vi "tree for Hardware Device Subpanel.vi"(1 "Data Types":T2(array[cluster]), 2 "Array":string[](array[string])=["Ring", "Elements", "to choose"], 3 "Data Names&Defaults":string[][](array[string])) -> (0 "Data Names&Data":string[][](array[string]))   [LabVIEW 2016, in "TSPopup.lvlib"]
doc: "Demo showing dynamically changing data types and working with a tree.\n\nType Sensitive Popup \nCopyright © 2007, J. David Saunders\nAll rights reserved."
uses:
  <userlib>/TSPopup/TSPopup.lvlib
  <userlib>/TSPopup/TSPopup.Popup Cluster.ctl
  <userlib>/TSPopup/TSPopup.lvclass
panel:
  in  "Array 2":string[](array[string])=["Ring", "Elements", "to choose"]
  in  "Remove Button":bool
  in  "Add Button":bool
  in  "Popups":T1 {"Boolean" items=["False", "True"]; "Ring" items=["Ring", "Elements", "to choose"]}
  in  "Cancel Button":bool
  in  "OK Button":bool
  in  "Data List":string(tree)
  # "Type Sensitive Popup \nCopyright © 2007, J. David Saunders\nAll rights reserved."
  # "Type Sensitive\nPopup"
  # "Boolean Colors"
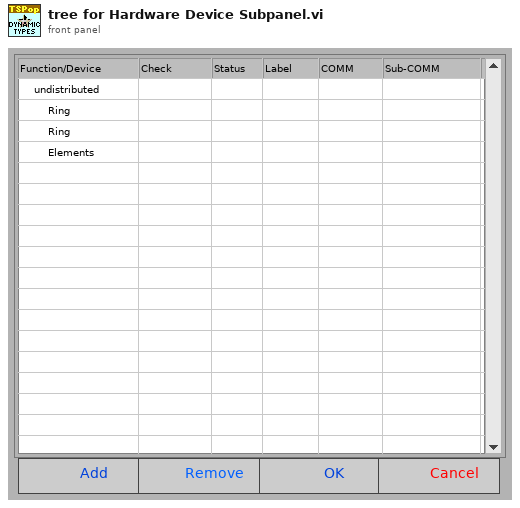
[diagram p1: front panel]
types:
  T1 = typedef "TSPopup.lvlib/TSPopup.lvclass/TSPopup.Popup Cluster.ctl" = cluster{"Unknown":bool, "Unknown 2":bool, "String":string, "Integer":i32, "Float":dbl, "Color":u32, "Boolean":u32, "Ring":u32, "Captioned String":cluster{"String":string, "OK":bool, "Cancel":bool}, "Captioned Integer":cluster{"First":i32, "OK":bool, "Cancel":bool}, "Boolean Colors":cluster{"False":cluster{"FG":u32, "BG":u32}, "True":cluster{"FG":u32, "BG":u32}, "T  to  F":cluster{"FG":u32, "BG":u32}, "F  to  T":cluster{"FG":u32, "BG":u32}, "OK":bool, "Cancel":bool}, "2-Int Cluster":cluster{"First":i32, "Second":i32, "OK":bool, "Cancel":bool}, "4-Int Cluster":cluster{"First":i32, "Second":i32, "Third":i32, "Fourth":i32, "OK":bool, "Cancel":bool}, "check":bool}
  T2 = cluster{"Data Type":string, "Caption/Ring Strings":string[]}[]
  T3 = typedef "LVPoint32TypeDef.ctl" = cluster{"Horizontal":i32, "Vertical":i32}
  T4 = typedef "TSPopup.lvlib/TSPopup.lvclass/TSPopup.Grid.Cell Info.ctl" = cluster{"Tag":string, "Row":i32, "Column":i32, "In Symbol?":bool, "In Data?":bool, "Cell String":string, "Ctl Refnum":refnum<vi>, "Prop Type":T5, "Ring Strings":string[]}
  T5 = typedef "TSPopup.lvlib/TSPopup.lvclass/TSPopup.Data Type.ctl" = enum16{"Unkown", "NO POPUP", "String", "Integer", "Float", "Color", "Boolean", "Ring", "Captioned String", "Captioned Integer", "Button Color", "2 Int Cluster", "4 Int Cluster", "check"}
  T6 = typedef "TSPopup.lvlib/TSPopup.lvclass/TSPopup.Popup Call Parameters.ctl" = cluster{"Prop Type":T5, "Initial Value":variant, "Caption Strings":string[], "Ring Strings":string[], "Cell Rect":cluster{"left":i16, "top":i16, "right":i16, "bottom":i16}, "Mouse Coords":cluster{"x":i16, "y":i16}, "Call Data":variant}
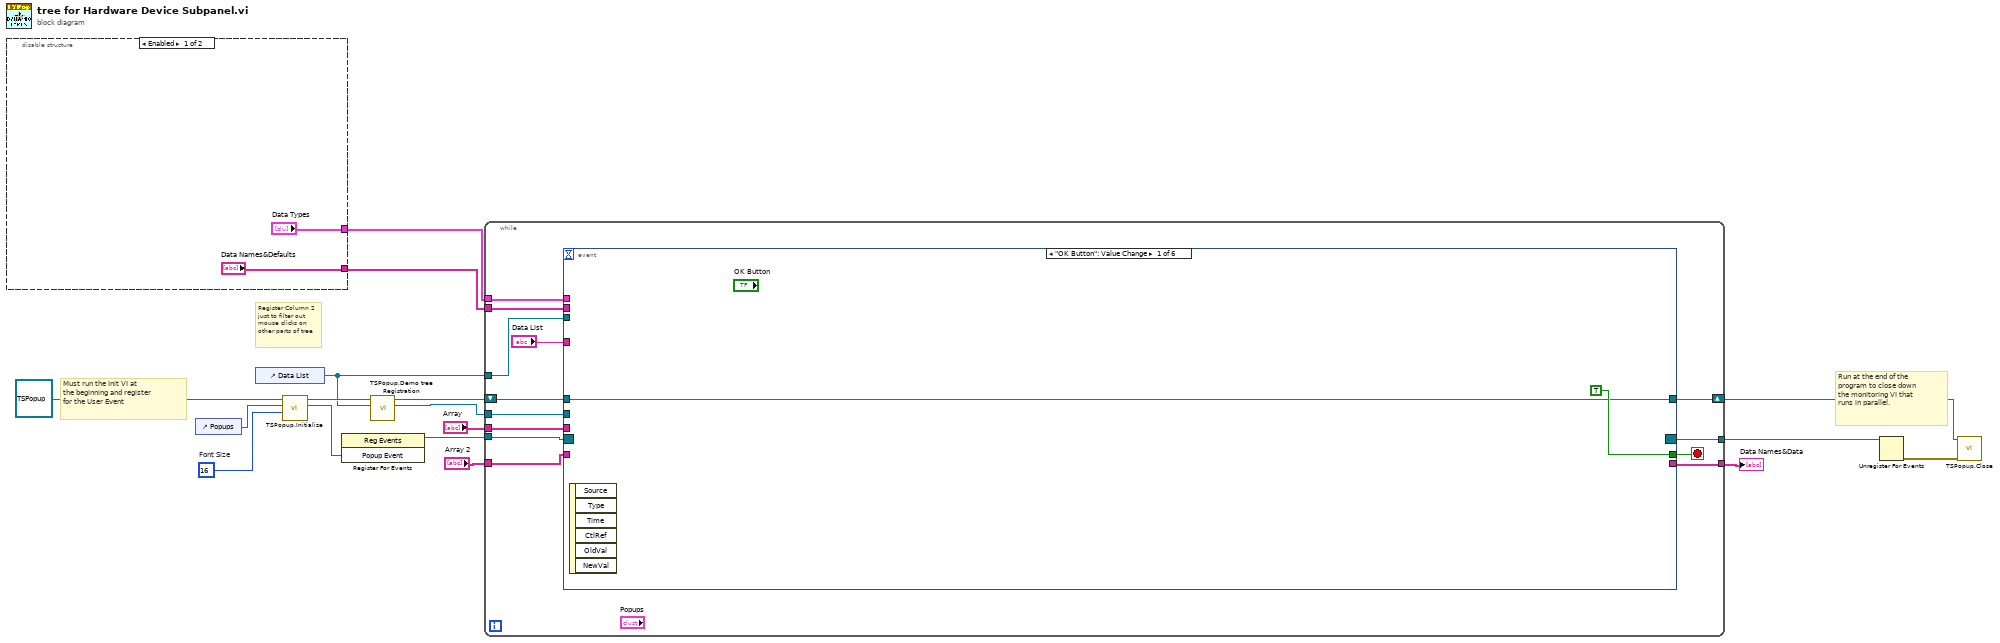
[diagram p0: block diagram]
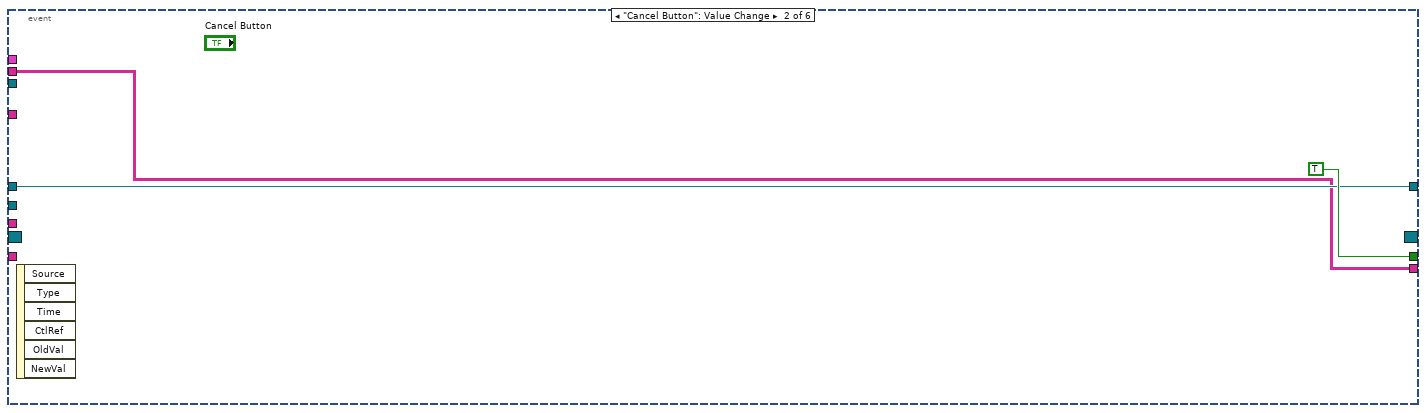
[diagram p2: hidden frame]
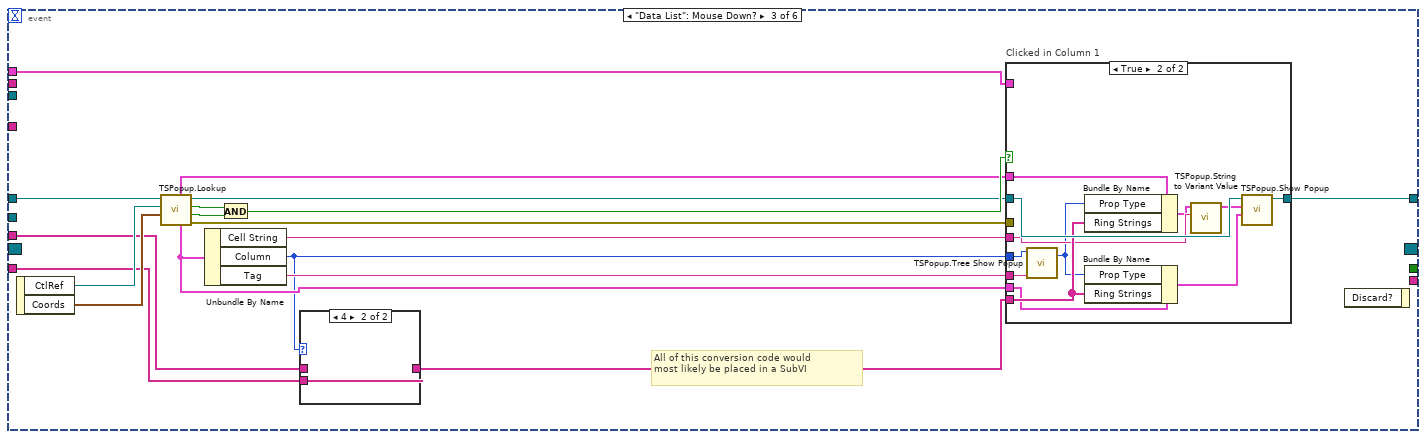
[diagram p3: hidden frame]
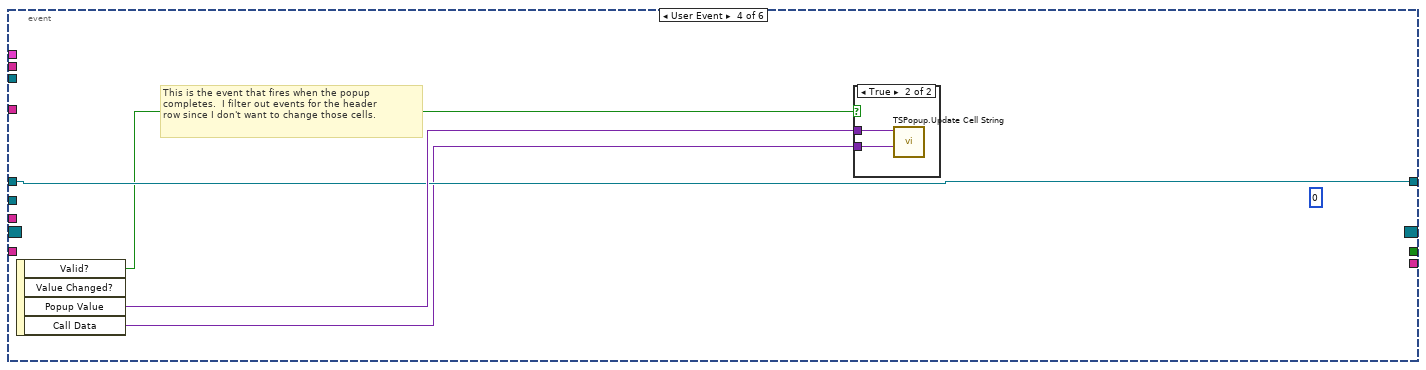
[diagram p6: hidden frame]
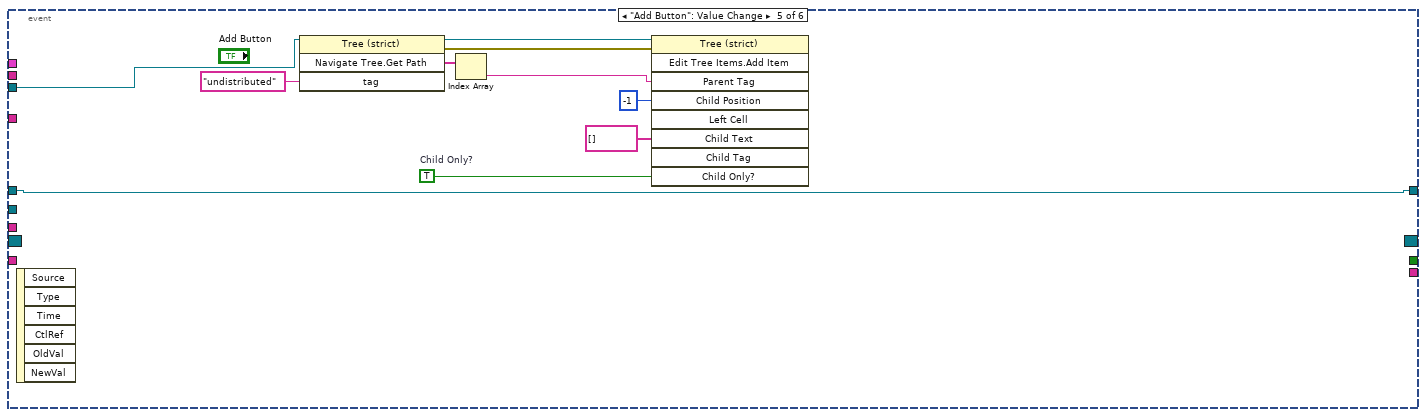
[diagram p8: hidden frame]
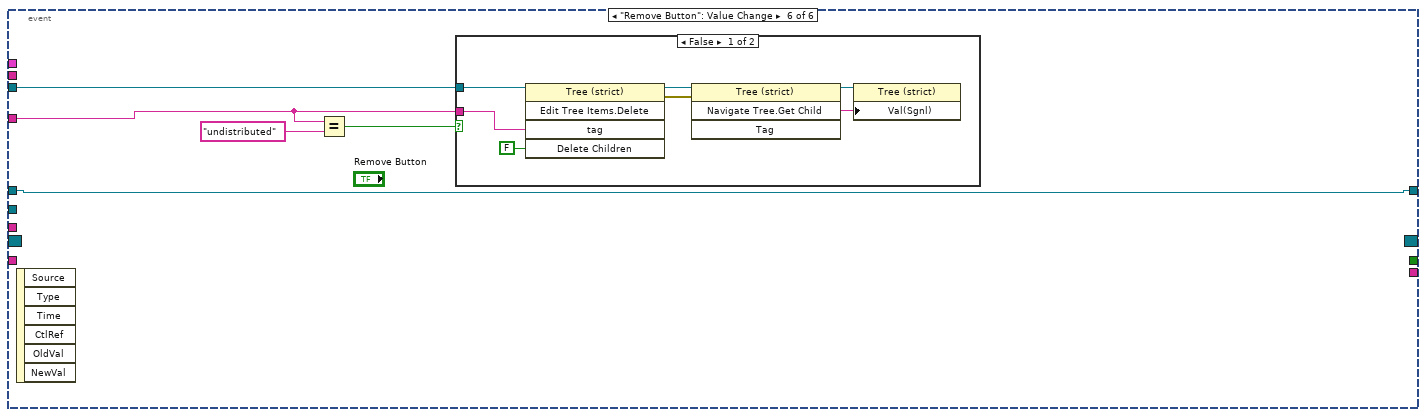
[diagram p9: hidden frame]
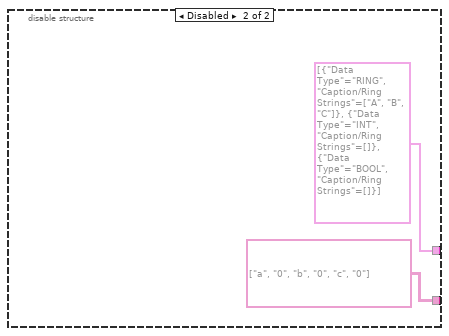
[diagram p11: hidden frame]
diagram:
  w13 = u32 16  # Font Size
  # "Register Column 2\njust to filter out\nmouse clicks on\nother parts of tree"
  # "Run at the end of the\nprogram to close down\nthe monitoring VI that\nruns in parallel."
  # "Must run the Init VI at\nthe beginning and register\nfor the User Event"
  n1 = disable-structure shown="Enabled" {
    disable-tunnel: ["Data Types" T2 [{"Data Type"="RING", "Caption/Ring Strings"=["A", "B", "C"]}, {"Data Type"="INT", "Caption/Ring Strings"=[]}, {"Data Type"="BOOL", "Caption/Ring Strings"=[]}] ("Data Types")] -> w7
    disable-tunnel: ["Data Names&Defaults" string[][] [["a", "0"], ["b", "0"], ["c", "0"]] ("Data Names&Defaults")] -> w8
    frame Enabled {
    }
    frame Disabled {
    }
  }
  n2 = control-ref of="Popups"() -> (w10:refnum<vi>)
  n3 = control-ref of="Data List"() -> (w2:refnum<vi>)
  n4 = call <userlib>:"TSPopup.Initialize.vi"("Font Size"=w13, "Popup Cluster Ref"=w10, "TSPopup in"=refnum<class "TSPopup.lvclass"> refnum ("TSPopup.lvclass")) -> ("Popup Event"=w12:refnum<user-event>, "TSPopup out"=w5:refnum<class "TSPopup.lvclass">)  [unwired: 6 in, 1 out]
  n5 = register-events(w12) -> (reference out=w17:refnum<event-registration>)  [unwired: 2 in, 1 out]
  n6 = call <userlib>:"TSPopup.Demo tree Registration.vi"("TSPopup in"=w5, "Signal Settings ref"=w2) -> ("TSPopup out"=w4:refnum<class "TSPopup.lvclass">, "dup ref out"=w3:refnum<vi>)  [unwired: 5 in, 1 out]
  n7 = while {
    tunnel: w17 -> [w34]
    tunnel: [w33] -> w16
    tunnel: w7 -> [w31]
    shift-right: [w29] -> w11
    shift-left: w4 -> [w30]
    tunnel: [w28] -> w9
    tunnel: w8 -> [w27]
    tunnel: "Array" -> [w26]
    tunnel: w3 -> [w25]
    tunnel: w2 -> [w23]
    tunnel: "Array 2" -> [w22]
    stop <- w32 stop-if-true
    n8 = event shown="[0] \"OK Button\": Value Change" {
      selector: w34 -> [_ _ _ _ _ _]
      dyn-events: [_ _ _ _ _ _] -> w33
      timeout: _ -> [_ _ _ _ _ _]
      tunnel: [TRUE TRUE _ _ _ _] -> w32
      tunnel: w31 -> [_ _ w56 _ _ _]
      tunnel: w30 -> [w35 w38 w49 w75 w88 w93]
      tunnel: [w35 w38 w47 w75 w88 w93] -> w29
      tunnel: [_ w37 _ _ _ _] -> w28
      tunnel: w27 -> [_ w37 _ _ _ _]
      tunnel: w26 -> [_ _ w42 _ _ _]
      tunnel: w25 -> [_ _ _ _ _ _]
      tunnel: w23 -> [_ _ _ _ w82 w89]
      tunnel: "Data List" -> [_ _ _ _ _ w90]
      tunnel: w22 -> [_ _ w41 _ _ _]
      event "OK Button": Value Change {
        n9 = event-data() -> ()  [unwired: 1 in, 6 out]
      }
      event "Cancel Button": Value Change {
        n10 = event-data() -> ()  [unwired: 1 in, 6 out]
      }
      event "Data List": Mouse Down? {
        # "All of this conversion code would\nmost likely be placed in a SubVI"
        n11 = event-data() -> ("CtlRef"=w55:refnum<vi>, "Coords"=w54:T3)  [unwired: 1 in]
        n12 = call <userlib>:"TSPopup.Lookup.vi"("Point"=w54, "Ctl Refnum"=w55, "TSPopup in"=w49) -> ("error out"=w50:errorcluster, "In Bounds?"=w51:bool, "Found"=w52:bool, "TSPopup out"=w48:refnum<class "TSPopup.lvclass">, "Cell Info (Call data)"=w46:T4, "Popup Parameters"=w53:T6)  [unwired: 3 in]
        n13 = Unbundle By Name(w46) -> ("Cell String"=w45:string, "Column"=w43:i32, "Tag"=w44:string)
        n14 = And(x=w52, y=w51) -> (x .and. y?=w57:bool)
        n15 = case shown="4" w43 {
          tunnel: w42 -> [w58 _]
          tunnel: w41 -> [_ w59]
          tunnel: [w58 w59] -> w40
          frame 0, Default {
          }
          frame 4 {
          }
        }
        n16 = case "Clicked in Column 1" shown="True" w57 {
          tunnel: w53 -> [_ w68]
          tunnel: w50 -> [_ _]
          tunnel: w56 -> [_ _]
          tunnel: w48 -> [w60 w72]
          tunnel: [w60 w71] -> w47
          tunnel: w46 -> [_ w65]
          tunnel: w45 -> [_ w69]
          tunnel: w40 -> [_ w70]
          tunnel: w43 -> [_ w63]
          tunnel: w44 -> [_ w61]
          frame False {
          }
          frame True {
            n17 = call <userlib>:"TSPopup.Tree Show Popup.vi"("Numeric"=w63, "String"=w61) -> ("Prop Type"=w62:T5)  [unwired: 4 in]
            n18 = Bundle By Name(cluster=w68, "Prop Type"=w62, "Ring Strings"=w70) -> (w67:T6)
            n19 = Bundle By Name(cluster=w65, "Prop Type"=w62, "Ring Strings"=w70) -> (w64:T4)
            n20 = call <userlib>:"TSPopup.String to Variant Value.vi"("Cell String"=w69, "Popup Parameters"=w67) -> ("Popup Parameters out"=w66:T6)  [unwired: 7 in, 2 out]
            n21 = call <userlib>:"TSPopup.Show Popup.vi"("Call Data (ignore if empty)"=w64, "Popup Parameters"=w66, "TSPopup in"=w72) -> ("TSPopup out"=w71:refnum<class "TSPopup.lvclass">)  [unwired: 7 in, 1 out]
          }
        }
        n22 = event-data() -> ()  [unwired: 2 in, 1 out]
      }
      event User Event {
        (unwired) 0 ("lower limit")
        # "This is the event that fires when the popup\ncompletes.  I filter out events for the header\nrow since I don't want to change those cells."
        n23 = event-data() -> ("Valid?"=w73:bool, "Popup Value"=w76:variant, "Call Data"=w74:variant)  [unwired: 1 in, 1 out]
        n24 = case shown="True" w73 {
          tunnel: w76 -> [_ w77]
          tunnel: w74 -> [_ w78]
          frame False {
          }
          frame True {
            n25 = call <userlib>:"TSPopup.Update Cell String.vi"("Call Data (must be Cell Info cluster)"=w78, "Popup Value"=w77) -> ()  [unwired: 9 in, 1 out]
          }
        }
      }
      event "Add Button": Value Change {
        w83 = TRUE  # Child Only?
        n26 = event-data() -> ()  [unwired: 1 in, 6 out]
        n27 = invoke on="Invoke Node" class="Tree (strict)" method="Navigate Tree.Get Path"(reference=w82, "tag"="undistributed" ("Tag")) -> (reference out=w81:refnum<vi>, error out=w86:errorcluster, "Navigate Tree:Get Path"=w87:string[])  [unwired: 2 in, 1 out]
        n28 = Index Array(array=w87) -> (element=w85:string)  [unwired: 1 in]
        n29 = invoke on="Invoke Node" class="Tree (strict)" method="Edit Tree Items.Add Item"(reference=w81, error in=w86, "Parent Tag"=w85, "Child Position"=-1, "Child Text"=string[] [], "Child Only?"=w83) -> ()  [unwired: 3 in, 9 out]
      }
      event "Remove Button": Value Change {
        n30 = event-data() -> ()  [unwired: 1 in, 6 out]
        n31 = Equal?(x=w90, y="undistributed" ("Tag")) -> (x = y?=w92:bool)
        n32 = case shown="False" w92 {
          tunnel: w89 -> [w98 _]
          tunnel: w90 -> [w95 _]
          frame False {
            n33 = invoke on="Invoke Node" class="Tree (strict)" method="Edit Tree Items.Delete"(reference=w98, "tag"=w95, "Delete Children"=FALSE ("Delete Children?")) -> (reference out=w97:refnum<vi>, error out=w99:errorcluster)  [unwired: 2 in, 3 out]
            n34 = invoke on="Invoke Node" class="Tree (strict)" method="Navigate Tree.Get Child"(reference=w97, error in=w99) -> (reference out=w96:refnum<vi>, "Navigate Tree:Get Child"=w100:string)  [unwired: 2 in, 2 out]
            n35 = property on="Property Node" class="Tree (strict)"(reference=w96, "Val(Sgnl)"=w100) -> ()  [unwired: 1 in, 2 out]
          }
          frame True {
          }
        }
      }
    }
  }
  "Data Names&Data" <- w9
  n36 = Unregister For Events(event registration refnum=w16) -> (error out=w15:errorcluster)  [unwired: 1 in]
  n37 = call <userlib>:"TSPopup.Close.vi"("error in (no error)"=w15, "TSPopup in"=w11) -> ()  [unwired: 8 in, 2 out]
